vi "LoggingHeaders.vi"(7 "Match Number":u32, 8 "error in":errorcluster, 9 "Battery Number":string, 10 "Date and Time":string, 11 "refnum in":refnum<file>) -> (0 "error out":errorcluster, 3 "refnum out":refnum<file>)   [LabVIEW 2017]
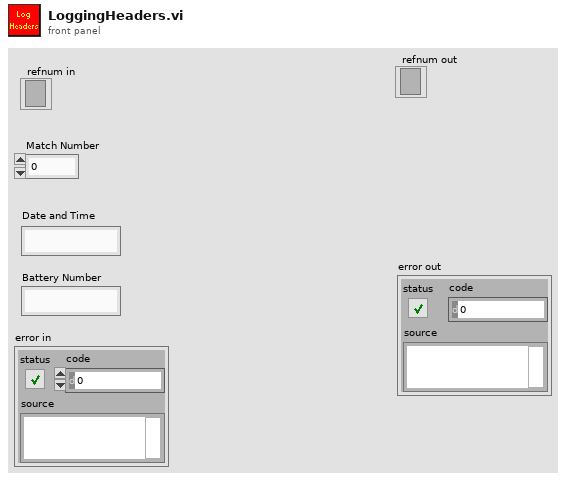
[diagram p1: front panel]
types:
  T1 = typedef "NetComm_MatchType.ctl" = enum32{"None", "Practice", "Qualification", "Elimination"}
  T2 = typedef "WPI_DriverStationPositionInfo.ctl" = enum16{"1", "2", "3"}
  T3 = typedef "WPI_DriverStationAllianceInfo.ctl" = enum16{"Red", "Blue", "Invalid"}
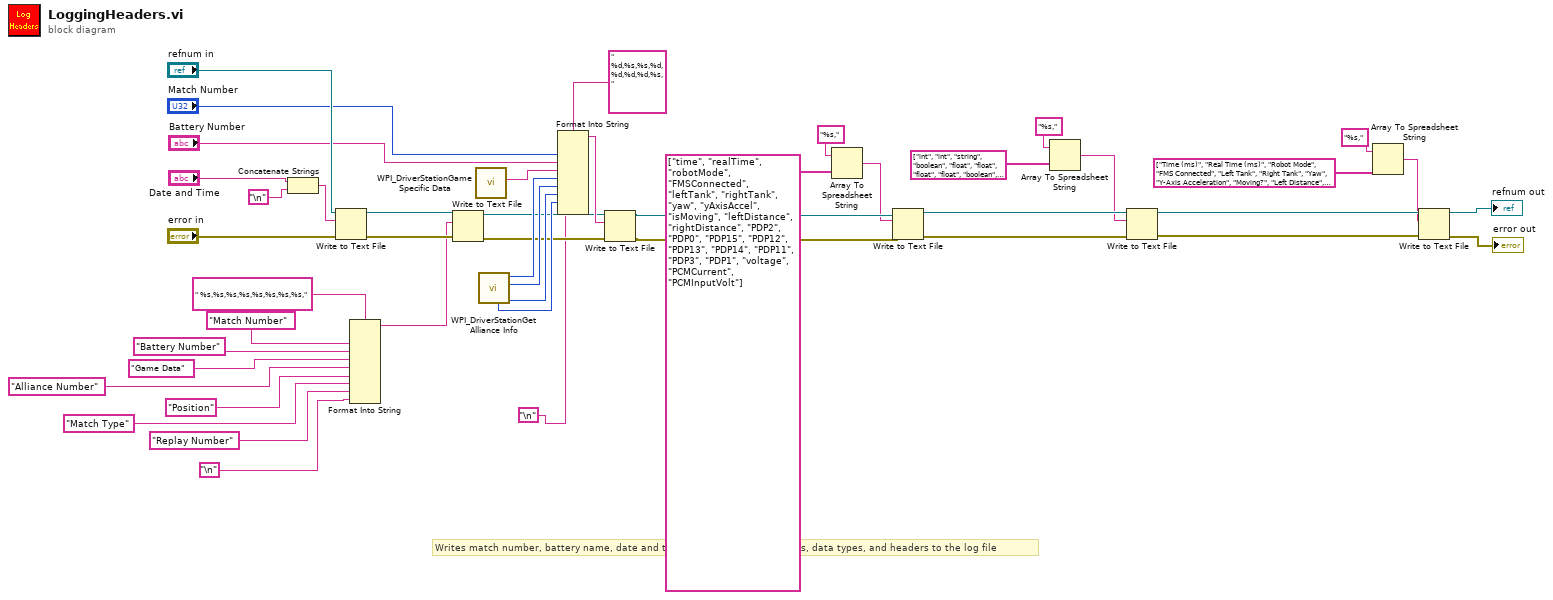
[diagram p0: block diagram]
diagram:
  # "Writes match number, battery name, date and time, headers variable names, data types, and headers to the log file"
  n1 = Concatenate Strings("Date and Time", "\n") -> (w44:string)
  n2 = Write to Text File(file (use dialog)="refnum in", text=w44, error in="error in") -> (refnum out=w15:refnum<file>, error out=w14:errorcluster)  [unwired: 1 in, 1 out]
  n3 = Format Into String(format string=" %s,%s,%s,%s,%s,%s,%s,%s,", "Match Number" ("input 2"), "Battery Number" ("input 2"), "Game Data" ("input 2"), "Alliance Number" ("input 2"), "Position" ("input 2"), "Match Type" ("input 2"), "Replay Number" ("input 2"), "\n") -> (resulting string=w3:string)  [unwired: 2 in, 1 out]
  n4 = Write to Text File(file (use dialog)=w15, text=w3, error in=w14) -> (refnum out=w12:refnum<file>, error out=w13:errorcluster)  [unwired: 1 in, 1 out]
  n5 = call <vilib>:"WPI_DriverStationGame Specific Data.vi"() -> ("Game Specific Data"=w20:string)  [unwired: 11 in]
  n6 = call <vilib>:"WPI_DriverStationGet Alliance Info.vi"() -> ("Match Type"=w17:T1, "Position"=w18:T2, "Alliance"=w19:T3, "Replay Number"=w16:u16)  [unwired: 6 in, 2 out]
  n7 = Format Into String(format string=" %d,%s,%s,%d,%d,%d,%d,%s,", "Match Number", "Battery Number", w20, w19, w18, w17, w16, "\n") -> (resulting string=w40:string)  [unwired: 2 in, 1 out]
  n8 = Write to Text File(file (use dialog)=w12, text=w40, error in=w13) -> (refnum out=w33:refnum<file>, error out=w32:errorcluster)  [unwired: 1 in, 1 out]
  n9 = Array To Spreadsheet String(array=string[] ["time", "realTime", "robotMode", "FMSConnected", "leftTank", "rightTank", "yaw", "yAxisAccel", "isMoving", "leftDistance", "rightDistance", "PDP2", "PDP0", "PDP15", "PDP12", "PDP13", "PDP14", "PDP11", "PDP3", "PDP1", "voltage", "PCMCurrent", "PCMInputVolt"], 3:"%s," ("format string")) -> (spreadsheet string=w25:string)  [unwired: 1 in]
  n10 = Write to Text File(file (use dialog)=w33, text=w25, error in=w32) -> (refnum out=w35:refnum<file>, error out=w34:errorcluster)  [unwired: 1 in, 1 out]
  n11 = Array To Spreadsheet String(array=string[] ["int", "int", "string", "boolean", "float", "float", "float", "float", "boolean", "float", "float", "float", "float", "float", "float", "float", "float", "float", "float", "float", "float", "float", "float"], 3:"%s," ("format string")) -> (spreadsheet string=w24:string)  [unwired: 1 in]
  n12 = Write to Text File(file (use dialog)=w35, text=w24, error in=w34) -> (refnum out=w29:refnum<file>, error out=w28:errorcluster)  [unwired: 1 in, 1 out]
  n13 = Array To Spreadsheet String(array=string[] ["Time (ms)", "Real Time (ms)", "Robot Mode", "FMS Connected", "Left Tank", "Right Tank", "Yaw", "Y-Axis Acceleration", "Moving?", "Left Distance", "Right Distance", "PWM 0 PDP 2 (L Drive)", "PWM 3 PDP 0 (L Drive)", "PWM 4 PDP 15 (L Drive)", "PWM 5 PDP 12 (R Drive)", "PWM 6 PDP 13 (R Drive)", "PWM 7 PDP 14 (R Drive)", "PWM 2 PDP 11 (Intake)", "PWM 1 PDP 3 (Scaler)", "PWM  9 PDP 1 (Scaler 2)", "Voltage", "PCM Current", "PCM Input Voltage"], 3:"%s," ("format string")) -> (spreadsheet string=w23:string)  [unwired: 1 in]
  n14 = Write to Text File(file (use dialog)=w29, text=w23, error in=w28) -> (refnum out=→"refnum out":refnum<file>, error out=→"error out":errorcluster)  [unwired: 1 in, 1 out]
